vi "turret speed.vi"(2 "rate in (-1 to 1)":dbl, 3 "Current Rate":dbl) -> (0 "output speed":dbl, 1 "current filtered rate":dbl format="%.2f")   [LabVIEW 2011]
uses:
  subStates.ctl
  <vilib>/addons/control/pid/pid.llb/PID Control Input Filter (DBL).vi
  <vilib>/addons/control/pid/pid.llb/PID (DBL).vi
  <vilib>/addons/control/pid/NI_PID_pid.lvlib
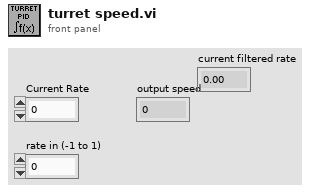
[diagram p1: front panel]
types:
  T1 = typedef "subStates.ctl" = enum16{"null", "wait", "driver control", "auto", "manual override", "autoDrive", "hold position", "rotate", "end"}
  T2 = cluster{"proportional gain (Kc)":dbl, "integral time (Ti, min)":dbl, "derivative time (Td, min)":dbl}
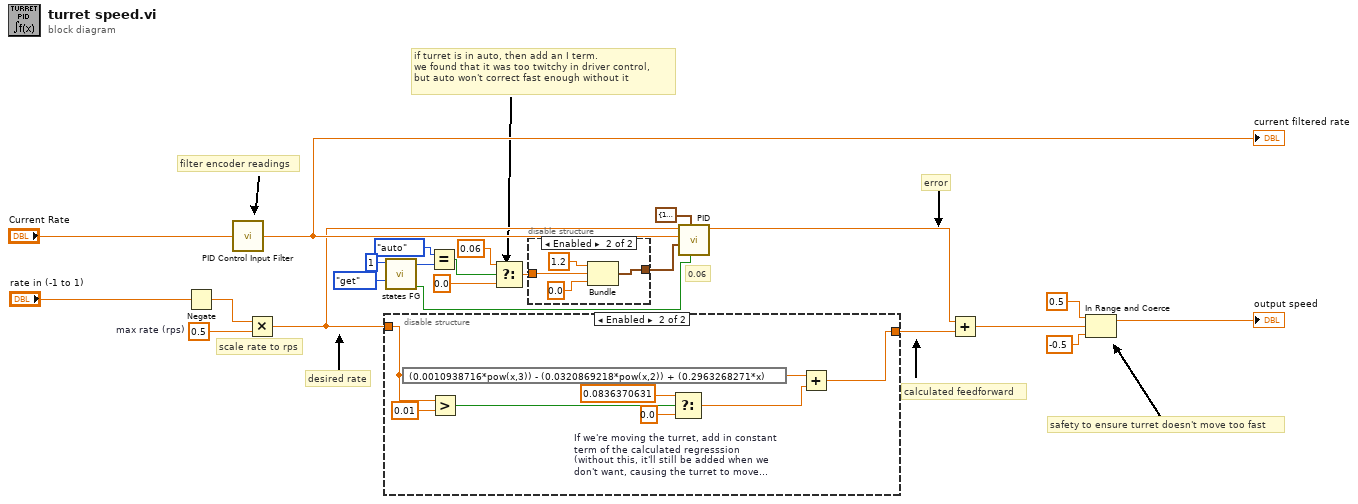
[diagram p0: block diagram]
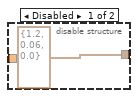
[diagram p2: hidden frame]
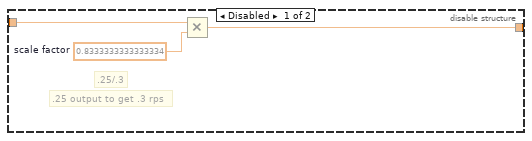
[diagram p3: hidden frame]
diagram:
  w13 = 0.5  # max rate (rps)
  # "if turret is in auto, then add an I term.\nwe found that it was too twitchy in driver control,\nbut auto won't correct fast enough without it"
  # "0.06"
  # "calculated feedforward"
  # "error"
  # "desired rate"
  # "filter encoder readings"
  # "scale rate to rps"
  # "safety to ensure turret doesn't move too fast"
  n1 = Negate(x="rate in (-1 to 1)") -> (-x=w21:dbl)
  n2 = call-poly <vilib>:"PID Control Input Filter.vi"("input"="Current Rate") -> ("output"=w15:dbl)  [unwired: 4 in]
  "current filtered rate" <- w15
  n3 = Multiply(x=w21, y=w13) -> (x*y=w14:dbl)
  n4 = disable-structure shown="Enabled" {
    disable-tunnel: [w25 w33] -> w18
    disable-tunnel: w14 -> [w24 w32]
    frame Disabled {
      w26 = 0.8333333333333334  # scale factor
      # ".25 output to get .3 rps"
      # ".25/.3"
      n5 = Multiply(x=w24, y=w26) -> (x*y=w25:dbl)
    }
    frame Enabled {
      n6 = expression code="(0.0010938716*pow(x,3)) - (0.0320869218*pow(x,2)) + (0.2963268271*x)"(w32) -> (w34:dbl)
      n7 = Greater?(x=w32, y=0.01) -> (0:w30:bool)
      n8 = Select "If we're moving the turret, add in constant\nterm of the calculated regresssion\n(without this, it'll still be added when we \ndon't want, causing the turret to move\nwhen it shouldn't)"(t=0.0836370631, s=w30, f=0.0) -> (s? t:f=w27:dbl)
      n9 = Add(x=w34, y=w27) -> (x+y=w33:dbl)
    }
  }
  n10 = call "states FG.vi"("menu (get)"=enum16{"set", "get"}."get", "Loop ID"=1) -> ("first call?"=w1:bool, "subState out"=w7:T1)  [unwired: 6 in, 2 out]
  n11 = Equal?(x=subStates."auto", y=w7) -> (x = y?=w5:bool)
  n12 = Select(t=0.06, s=w5, f=0.0) -> (s? t:f=w2:dbl)
  n13 = disable-structure shown="Enabled" {
    disable-tunnel: [T2 {"proportional gain (Kc)"=1.2, "integral time (Ti, min)"=0.06, "derivative time (Td, min)"=0.0} ("PID gains") w38] -> w17
    disable-tunnel: w2 -> [_ w39]
    frame Disabled {
    }
    frame Enabled {
      n14 = Bundle("f"=1.2, "f"=w39, "f"=0.0) -> (w38:cluster{"f":dbl, "f":dbl, "f":dbl})  [unwired: 1 in]
    }
  }
  n15 = call-poly <vilib>:"PID.vi"("reinitialize? (F)"=w1, "output range"=cluster{"output high":dbl, "output low":dbl} {"output high"=1.0, "output low"=-1.0}, "PID gains"=w17, "process variable"=w15, "setpoint"=w14) -> ("output"=w19:dbl)  [unwired: 5 in, 1 out]
  n16 = Add(x=w19, y=w18) -> (x+y=w20:dbl)
  n17 = In Range and Coerce(upper limit=0.5, x=w20, lower limit=-0.5) -> (coerced(x)=→"output speed":dbl)  [unwired: 1 out]
